vi "Events Cluster Label Text.vi"() -> (0 "Events Cluster Label Text":string)   [LabVIEW 2018, in "Scripting.lvlib"]
uses:
  Scripting.lvlib
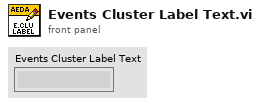
[diagram p1: front panel]
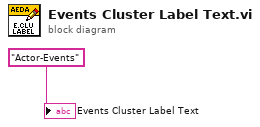
[diagram p0: block diagram]
diagram:
  "Events Cluster Label Text" <- "Actor-Events" ("y")
